vi "place in stack third row.vi"(8 "angle 2":i32, 9 "angle":i32, 10 "c2":dbl, 11 "c1":dbl) -> ()   [LabVIEW 2018]
uses:
  ARM angles.vi
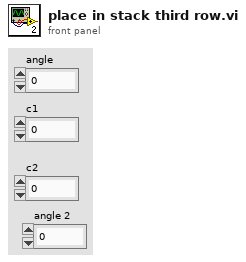
[diagram p1: front panel]
types:
  T1 = enum16{"shoulder", "elbow", "wrist", "base", "gripper"}
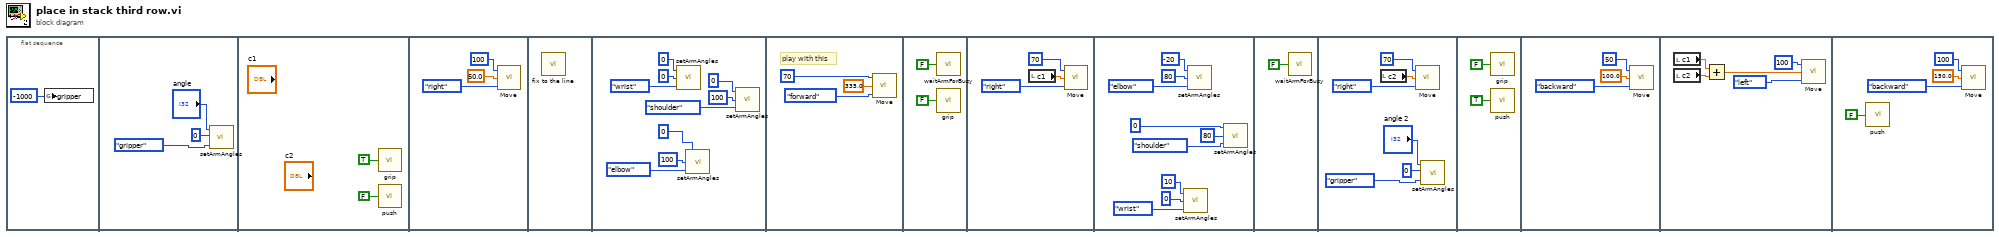
[diagram p0: block diagram]
diagram:
  n1 = flat-sequence {
    frame #0 {
      n2 = global write "ARM angles.vi" "gripper"(-1000 ("gripper")) -> ()
    }
    frame #1 {
      n3 = call "setArmAngles.vi"("Enum"=T1."gripper", "speed"=0, "angle"="angle") -> ()  [unwired: 1 in]
    }
    frame #2 {
      n4 = call "grip.vi"("grip"=TRUE) -> ()
      n5 = call "push.vi"("push"=FALSE) -> ()
    }
    frame #3 {
      n6 = call "Move.vi"("Enum"=enum16{"forward", "backward", "left", "right"}."right", "distance"=50.0, "speed"=100) -> ()  [unwired: 1 in]
    }
    frame #4 {
      n7 = call "fix to the line.vi"() -> ()  [unwired: 12 in]
    }
    frame #5 {
      n8 = call "setArmAngles.vi"("Enum"=T1."wrist", "speed"=0, "angle"=0) -> ()  [unwired: 1 in]
      n9 = call "setArmAngles.vi"("Enum"=T1."elbow", "speed"=100, "angle"=0) -> ()  [unwired: 1 in]
      n10 = call "setArmAngles.vi"("Enum"=T1."shoulder", "speed"=100, "angle"=0) -> ()  [unwired: 1 in]
    }
    frame #6 {
      # "play with this"
      n11 = call "Move.vi"("Enum"=enum16{"forward", "backward", "left", "right"}."forward", "distance"=335.0, "speed"=70) -> ()  [unwired: 1 in]
    }
    frame #7 {
      n12 = call "waitArmForBusy.vi"("base"=FALSE) -> ()
      n13 = call "grip.vi"("grip"=FALSE) -> ()
    }
    frame #8 {
      n14 = local read "c1"() -> (w24:dbl)
      n15 = call "Move.vi"("Enum"=enum16{"forward", "backward", "left", "right"}."right", "distance"=w24, "speed"=70) -> ()  [unwired: 1 in]
    }
    frame #9 {
      n16 = call "setArmAngles.vi"("Enum"=T1."wrist", "speed"=0, "angle"=10) -> ()  [unwired: 1 in]
      n17 = call "setArmAngles.vi"("Enum"=T1."elbow", "speed"=80, "angle"=-20) -> ()  [unwired: 1 in]
      n18 = call "setArmAngles.vi"("Enum"=T1."shoulder", "speed"=80, "angle"=0) -> ()  [unwired: 1 in]
    }
    frame #10 {
      n19 = call "waitArmForBusy.vi"("base"=FALSE) -> ()
    }
    frame #11 {
      n20 = local read "c2"() -> (w40:dbl)
      n21 = call "Move.vi"("Enum"=enum16{"forward", "backward", "left", "right"}."right", "distance"=w40, "speed"=70) -> ()  [unwired: 1 in]
      n22 = call "setArmAngles.vi"("Enum"=T1."gripper", "speed"=0, "angle"="angle 2") -> ()  [unwired: 1 in]
    }
    frame #12 {
      n23 = call "grip.vi"("grip"=FALSE) -> ()
      n24 = call "push.vi"("push"=TRUE) -> ()
    }
    frame #13 {
      n25 = call "Move.vi"("Enum"=enum16{"forward", "backward", "left", "right"}."backward", "distance"=100.0, "speed"=50) -> ()  [unwired: 1 in]
    }
    frame #14 {
      n26 = local read "c1"() -> (w50:dbl)
      n27 = local read "c2"() -> (w49:dbl)
      n28 = Add(x=w50, y=w49) -> (x+y=w48:dbl)
      n29 = call "Move.vi"("Enum"=enum16{"forward", "backward", "left", "right"}."left", "distance"=w48, "speed"=100) -> ()  [unwired: 1 in]
    }
    frame #15 {
      n30 = call "push.vi"("push"=FALSE) -> ()
      n31 = call "Move.vi"("Enum"=enum16{"forward", "backward", "left", "right"}."backward", "distance"=150.0, "speed"=100) -> ()  [unwired: 1 in]
    }
  }
